vi "FaceGrabber.vi"() -> ()   [LabVIEW 2020]
uses:
  <vilib>/Utility/file.llb/Write Delimited Spreadsheet (string).vi
  <vilib>/vision/NI_Vision_Development_Module.lvlib
panel:
  in  "new table":bool
  in  "open table":bool
  out "Categories":string[](array[string])=["grooming", "aggression", "monkey_play", "group", "mating", "baby_monkey", "animals_playing", "hiding"]
  out "All Files in Dir":path[](array[path])
  out "data":cluster{"pictures":path, "table":path}
  in  "delete object":bool
  out "output array":string[][](array[string])
  in  "Table with results":path=path "C:/YandexDisk/MonkeysDatas/data/out/stimuli_set_lnv/area.csv"
  in  "save all":bool
  out "contours":T1(array[cluster])
  in  "category":u16(ring) items=["grooming", "aggression", "monkey_play", "group", "mating", "baby_monkey", "animals_playing", "hiding"]
  in  "add object":bool
  out "number of pictures":i32=120
  out "picture":i32
  in  "Stimuli Folder Path":path=path "C:/YandexDisk/MonkeysDatas/data/stimuli_set_lnv"
  in  "stop":bool
  in  "previous":bool
  in  "next":bool
  out "Image":T2(plugin-control)
  in  "baby/adult":bool=TRUE
  in  "face":bool=TRUE
  in  "animal":bool
  in  "monkey":bool=TRUE
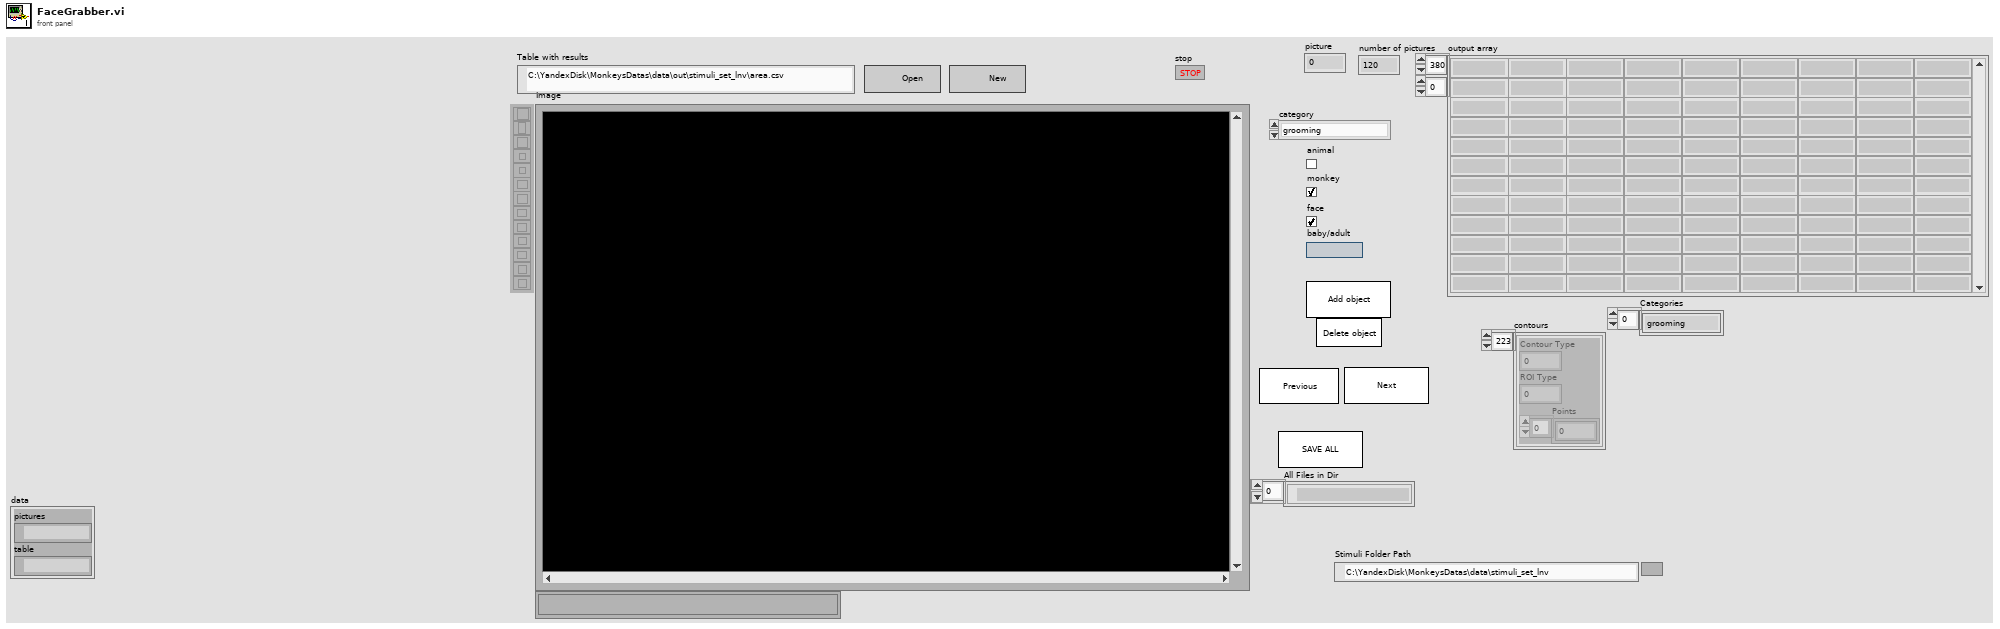
[diagram p1: front panel]
types:
  T1 = cluster{"Contour Type":u32, "ROI Type":u32, "Points":i32[]}[]
  T2 = typedef "IMAQ Image.ctl" = refnum<image>
  T3 = cluster{"stimuli pictures":path, "results table":path}
  T4 = cluster{"Stimuli Folder Path":path, "Table with results":path}
  T5 = cluster{"Global Rectangle":i32[], "Contours":cluster{"Contour Type":u32, "ROI Type":u32, "Points":i32[]}[]}
  T6 = typedef "Particle Parameters" = i32
  T7 = cluster{"Contour Type":u32, "ROI Type":u32, "Points":i32[]}
  T8 = cluster{"Stimuli Folder Path":path, "selected path":path}
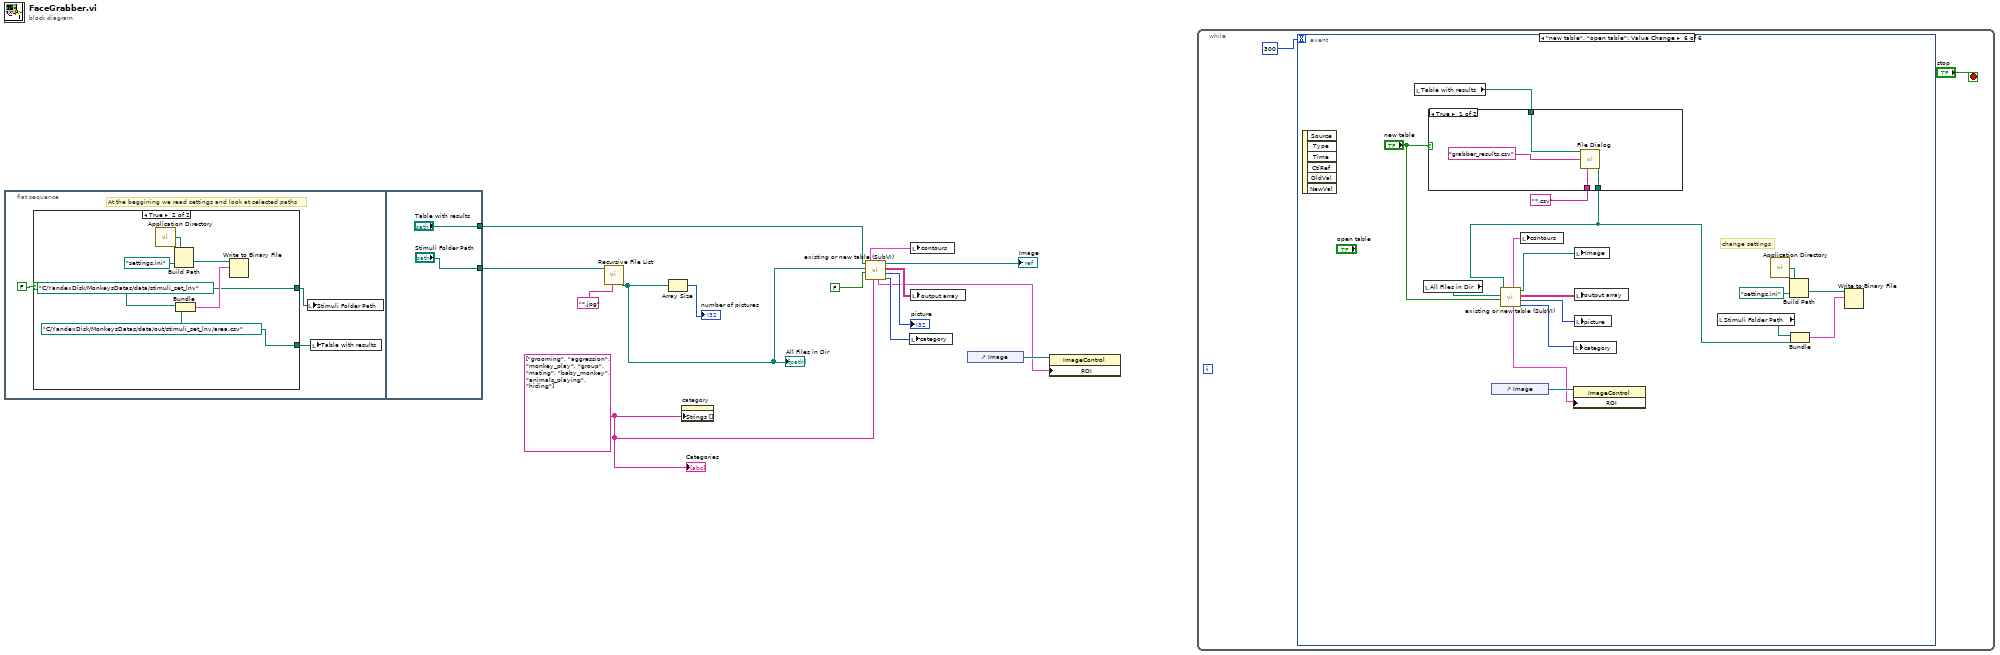
[diagram p0: block diagram]
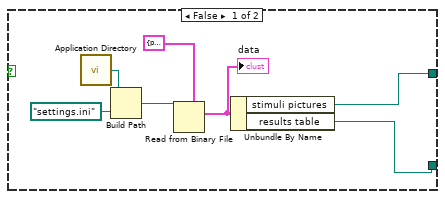
[diagram p2: hidden frame]
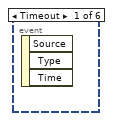
[diagram p3: hidden frame]
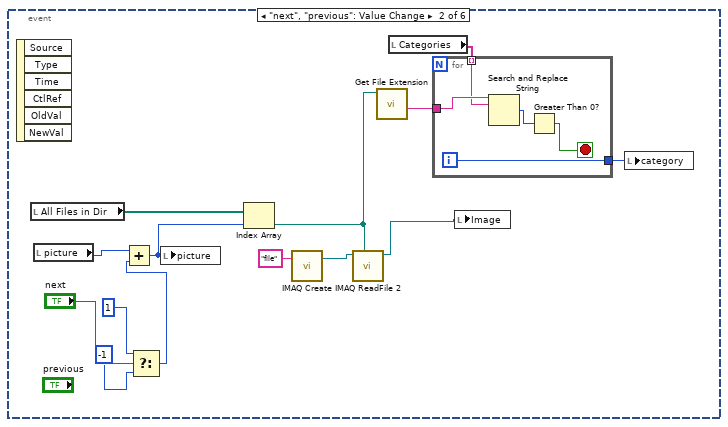
[diagram p4: hidden frame]
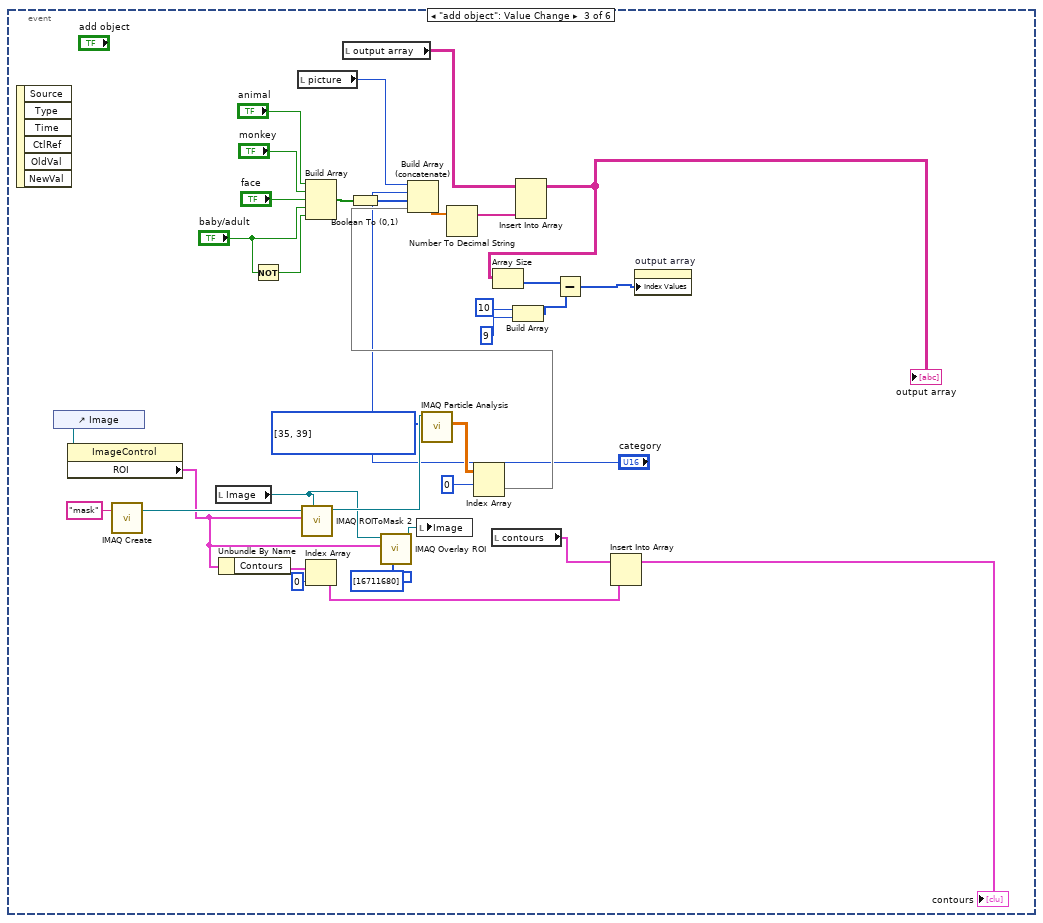
[diagram p5: hidden frame]
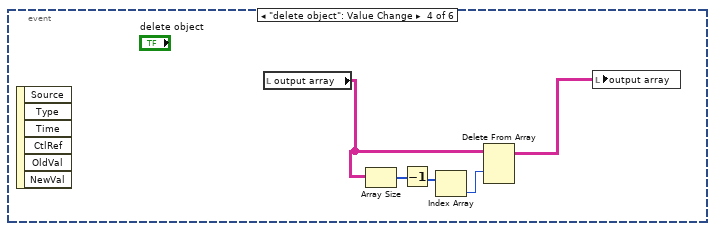
[diagram p6: hidden frame]
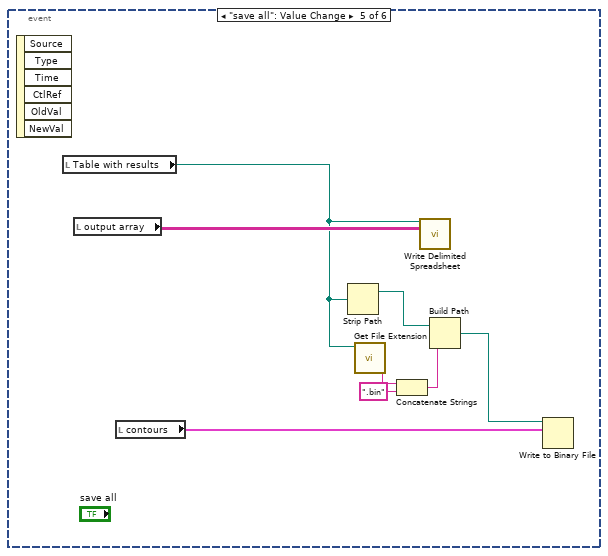
[diagram p7: hidden frame]
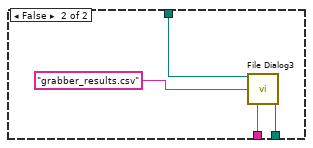
[diagram p8: hidden frame]
diagram:
  w3 = string[] ["grooming", "aggression", "monkey_play", "group", "mating", "baby_monkey", "animals_playing", "hiding"] ("Strings []")
  n1 = flat-sequence {
    tunnel: ["Table with results"] -> w2
    tunnel: ["Stimuli Folder Path"] -> w1
    frame #0 {
      # "At the beggining we read settings and look at selected paths"
      n2 = case shown="True" FALSE {
        tunnel: [w18 w26] -> w16
        tunnel: [w19 w25] -> w15
        frame False {
          n3 = call <vilib>:"Application Directory.vi"() -> ("Application Directory"=w22:path)
          n4 = Build Path(base path=w22, name or relative path=path "settings.ini") -> (appended path=w23:path)
          n5 = Read from Binary File(5:T3 {"stimuli pictures"=path "", "results table"=path ""} ("output cluster"), 11:w23) -> (2:w24:T3)  [unwired: 4 in, 3 out]
          "data" <- w24
          n6 = Unbundle By Name(w24) -> ("stimuli pictures"=w19:path, "results table"=w18:path)
        }
        frame True {
          w26 = path "C:/YandexDisk/MonkeysDatas/data/out/stimuli_set_lnv/area.csv" ("Table with results")
          w25 = path "C:/YandexDisk/MonkeysDatas/data/stimuli_set_lnv" ("Stimuli Folder Path")
          n7 = call <vilib>:"Application Directory.vi"() -> ("Application Directory"=w30:path)
          n8 = Build Path(base path=w30, name or relative path=path "settings.ini") -> (appended path=w28:path)
          n9 = Bundle("Stimuli Folder Path"=w25, "Table with results"=w26) -> (w27:T4)  [unwired: 1 in]
          n10 = Write to Binary File(file (use dialog)=w28, data=w27) -> ()  [unwired: 4 in, 3 out]
        }
      }
      n11 = local write "Stimuli Folder Path"(w15) -> ()
      n12 = local write "Table with results"(w16) -> ()
    }
    frame #1 {
    }
  }
  n13 = call <vilib>:"Recursive File List.vi"("pattern"="*.jpg", "Folder Path"=w1) -> ("All Files in Dir"=w4:path[])  [unwired: 5 in, 4 out]
  "All Files in Dir" <- w4
  n14 = Array Size(array=w4) -> (size(s)=→"number of pictures":i32)
  n15 = property on="category" class="Ring (strict)"("Strings []"=w3) -> ()  [unwired: 2 in, 2 out]
  n16 = call "existing or new table (SubVI).vi"("Categories (in)"=w3, "new table?"=FALSE, "All Files in Dir (in)"=w4, "table"=w2) -> ("category"=w6:i32, "picture"=→"picture":i32, "text table"=w7:string[][], "Refnum out"=→"Image":T2, "ROI"=w5:T5, "contours"=w8:T1)  [unwired: 2 in]
  n17 = local write "category"(w6) -> ()
  n18 = local write "contours"(w8) -> ()
  n19 = local write "output array"(w7) -> ()
  n20 = control-ref of="Image"() -> (w12:refnum<vi>)
  n21 = property class="ImageControl"(reference=w12, "ROI"=w5) -> ()  [unwired: 1 in, 2 out]
  n22 = while {
    stop <- "stop" stop-if-true
    n23 = event shown="[5] \"new table\", \"open table\": Value Change" {
      selector: _ -> [_ _ _ _ _ _]
      dyn-events: _ -> [_ _ _ _ _ _]
      timeout: 300 -> [_ _ _ _ _ _]
      event Timeout {
        n24 = event-data() -> ()  [unwired: 1 in, 3 out]
      }
      event "next", "previous": Value Change {
        n25 = event-data() -> ()  [unwired: 1 in, 6 out]
        n26 = local read "All Files in Dir"() -> (w37:path[])
        n27 = local read "picture"() -> (w36:i32)
        n28 = Select(t=1 ("y"), s="next", f=-1 ("y")) -> (s? t:f=w42:i32)
        n29 = Add(x=w36, y=w42) -> (x+y=w41:i32)
        n30 = local write "picture"(w41) -> ()
        n31 = Index Array(array=w37, index=w41) -> (element=w40:path)
        n32 = call "IMAQ Create"("Image Name"="file") -> ("New Image"=w48:T2)  [unwired: 4 in, 1 out]
        n33 = call "IMAQ ReadFile 2"("File Path"=w40, "Image"=w48) -> ("Image Out"=w46:T2)  [unwired: 5 in, 4 out]
        n34 = call <vilib>:"Get File Extension.vi"("file"=w40) -> ("filename without extension"=w39:string)  [unwired: 6 in, 4 out]
        n35 = local read "Categories"() -> (w35:string[])
        n36 = for {
          tunnel: w35 -> [w52] mode=indexing
          tunnel: w39 -> [w53]
          tunnel: [w49] -> w38
          i -> [w49]
          stop <- w50 stop-if-true
          n37 = Search and Replace String(input string=w53, search string=w52) -> (number of replacements=w51:i32)  [unwired: 6 in, 3 out]
          n38 = Greater Than 0?(x=w51) -> (x > 0?=w50:bool)
        }
        n39 = local write "Image"(w46) -> ()
        n40 = local write "category"(w38) -> ()
      }
      event "add object": Value Change {
        w79 = T6[] [35, 39] items=["Center of Mass X", "Center of Mass Y", "First Pixel X", "First Pixel Y", "Bounding Rect Left", "Bounding Rect Top", "Bounding Rect Right", "Bounding Rect Bottom", "Max Feret Diameter Start X", "Max Feret Diameter Start Y", "Max Feret Diameter End X", "Max Feret Diameter End Y", "Max Horiz. Segment Length Left", "Max Horiz. Segment Length Right", "Max Horiz. Segment Length Row", "-", "Bounding Rect Width", "Bounding Rect Height", "Bounding Rect Diagonal", "Perimeter", "Convex Hull Perimeter", "Holes' Perimeter", "Max Feret Diameter", "Equivalent Ellipse Major Axis", "Equivalent Ellipse Minor Axis", "Equivalent Ellipse Minor Axis (Feret)", "Equivalent Rect Long Side", "Equivalent Rect Short Side", "Equivalent Rect Diagonal", "Equivalent Rect Short Side (Feret)", "Average Horiz. Segment Length", "Average Vert. Segment Length", "Hydraulic Radius", "Waddel Disk Diameter", "-", "Area", "Holes' Area", "Particle & Holes' Area", "Convex Hull Area", "Image Area", "-", "Number of Holes", "Number of Horiz. Segments", "Number of Vert. Segments", "-", "Orientation", "Max Feret Diameter Orientation", "-", "% Area/Image Area", "% Area/(Particle & Holes' Area)", "Ratio of Equivalent Ellipse Axes", "Ratio of Equivalent Rect Sides", "-", "Elongation Factor", "Compactness Factor", "Heywood Circularity Factor", "Type Factor", "-", "Sum X", "Sum Y", "Sum XX", "Sum XY", "Sum YY", "Sum XXX", "Sum XXY", "Sum XYY", "Sum YYY", "-", "Moment of Inertia XX", "Moment of Inertia XY", "Moment of Inertia YY", "Moment of Inertia XXX", "Moment of Inertia XXY", "Moment of Inertia XYY", "Moment of Inertia YYY", "Norm. Moment of Inertia XX", "Norm. Moment of Inertia XY", "Norm. Moment of Inertia YY", "Norm. Moment of Inertia XXX", "Norm. Moment of Inertia XXY", "Norm. Moment of Inertia XYY", "Norm. Moment of Inertia YYY", "Hu Moment 1", "Hu Moment 2", "Hu Moment 3", "Hu Moment 4", "Hu Moment 5", "Hu Moment 6", "Hu Moment 7"] ("Pixel Measurements")
        n41 = event-data() -> ()  [unwired: 1 in, 6 out]
        n42 = control-ref of="Image"() -> (w77:refnum<vi>)
        n43 = property class="ImageControl"(reference=w77) -> ("ROI"=w59:T5)  [unwired: 1 in, 2 out]
        n44 = call "IMAQ Create"("Image Name"="mask") -> ("New Image"=w82:T2)  [unwired: 4 in, 1 out]
        n45 = local read "Image"() -> (w60:T2)
        n46 = Unbundle By Name(w59) -> ("Contours"=w76:T1)
        n47 = Not(x="baby/adult") -> (.not. x?=w55:bool)
        n48 = local read "picture"() -> (w54:i32)
        n49 = call "IMAQ ROIToMask 2"("Image Model"=w60, "ROI Descriptor"=w59, "Image"=w82) -> ("Image Out"=w83:T2)  [unwired: 6 in, 2 out]
        n50 = Build Array("animal", "monkey", "face", "baby/adult", w55) -> (w87:bool[])
        n51 = Index Array(array=w76, index=0) -> (element=w71:T7)
        n52 = local read "output array"() -> (w74:string[][])
        n53 = Boolean To (0,1)(Boolean=w87) -> (0, 1=w88:i16[])
        n54 = call "IMAQ Overlay ROI"("Colors (Green)"=u32[] [16711680], "ROI Descriptor"=w59, "Image"=w60) -> ("Image Out"=w58:T2)  [unwired: 7 in, 1 out]
        n55 = local write "Image"(w58) -> ()
        n56 = call "IMAQ Particle Analysis"("Pixel Measurements"=w79, "Image"=w83) -> ("Particle Measurements (Pixels)"=w81:dbl[][])  [unwired: 4 in, 5 out]
        n57 = Index Array(array=w81, index (row)=0 ("disabled index (col)")) -> (element=w78:dbl[])  [unwired: 1 in]
        n58 = Build Array (concatenate)(w54, "category", w88, w78) -> (w73:dbl[])
        n59 = Number To Decimal String(number=w73) -> (decimal integer string=w67:string[])  [unwired: 1 in]
        n60 = local read "contours"() -> (w69:T1)
        n61 = Build Array(10, 9) -> (w64:i32[])
        n62 = Insert Into Array(array=w74, new element=w67) -> (w66:string[][])  [unwired: 2 in]
        "output array" <- w66
        n63 = Array Size(array=w66) -> (size(s)=w65:i32[])
        n64 = Subtract(x=w65, y=w64) -> (x-y=w63:i32[])
        n65 = Insert Into Array(array=w69, new element=w71) -> (→"contours":T1)  [unwired: 1 in]
        n66 = property on="output array" class="Arr (strict)"("Index Values"=w63) -> ()  [unwired: 2 in, 2 out]
      }
      event "delete object": Value Change {
        n67 = event-data() -> ()  [unwired: 1 in, 6 out]
        n68 = local read "output array"() -> (w90:string[][])
        n69 = Array Size(array=w90) -> (size(s)=w91:i32[])
        n70 = Decrement(x=w91) -> (x-1=w92:i32[])
        n71 = Index Array(array=w92) -> (element=w93:i32)  [unwired: 1 in]
        n72 = Delete From Array(array=w90, index (row)=w93) -> (array with subset deleted=w89:string[][])  [unwired: 2 in, 1 out]
        n73 = local write "output array"(w89) -> ()
      }
      event "save all": Value Change {
        n74 = event-data() -> ()  [unwired: 1 in, 6 out]
        n75 = local read "Table with results"() -> (w94:path)
        n76 = local read "output array"() -> (w95:string[][])
        n77 = local read "contours"() -> (w101:T1)
        n78 = Strip Path(path=w94) -> (stripped path=w97:path)  [unwired: 1 out]
        n79 = call <vilib>:"Get File Extension.vi"("file"=w94) -> ("filename without extension"=w100:string)  [unwired: 6 in, 4 out]
        n80 = Concatenate Strings(w100, ".bin" ("string")) -> (w98:string)
        n81 = call-poly <vilib>:"Write Delimited Spreadsheet.vi"("file path (dialog if empty)"=w94, "2D data"=w95) -> ()  [unwired: 12 in, 2 out]
        n82 = Build Path(base path=w97, name or relative path=w98) -> (appended path=w96:path)
        n83 = Write to Binary File(file (use dialog)=w96, data=w101) -> ()  [unwired: 4 in, 3 out]
      }
      event "new table", "open table": Value Change {
        # "change settings"
        n84 = event-data() -> ()  [unwired: 1 in, 6 out]
        n85 = local read "Table with results"() -> (w109:path)
        n86 = local read "All Files in Dir"() -> (w110:path[])
        n87 = case shown="True" "new table" {
          tunnel: [w122 w126] -> w102
          tunnel: w109 -> [w120 w124]
          tunnel: "*.csv" ("pattern (all files)") -> [w119 w123]
          frame True {
            n88 = call "File Dialog"("start path"=w120, "default name"="grabber_results.csv", "pattern (all files)"=w119) -> ("selected path"=w122:path)  [unwired: 9 in, 3 out]
          }
          frame False {
            n89 = call "File Dialog3"("start path"=w124, "default name"="grabber_results.csv", "pattern (all files)"=w123) -> ("selected path"=w126:path)  [unwired: 9 in, 3 out]
          }
        }
        n90 = control-ref of="Image"() -> (w107:refnum<vi>)
        n91 = call "existing or new table (SubVI).vi"("new table?"="new table", "All Files in Dir (in)"=w110, "table"=w102) -> ("category"=w112:i32, "picture"=w113:i32, "text table"=w114:string[][], "Refnum out"=w111:T2, "ROI"=w106:T5, "contours"=w105:T1)  [unwired: 3 in]
        n92 = local write "contours"(w105) -> ()
        n93 = local write "category"(w112) -> ()
        n94 = property class="ImageControl"(reference=w107, "ROI"=w106) -> ()  [unwired: 1 in, 2 out]
        n95 = local write "output array"(w114) -> ()
        n96 = local write "picture"(w113) -> ()
        n97 = local write "Image"(w111) -> ()
        n98 = local read "Stimuli Folder Path"() -> (w103:path)
        n99 = call <vilib>:"Application Directory.vi"() -> ("Application Directory"=w115:path)
        n100 = Build Path(base path=w115, name or relative path=path "settings.ini") -> (appended path=w117:path)
        n101 = Bundle("Stimuli Folder Path"=w103, "selected path"=w102) -> (w118:T8)  [unwired: 1 in]
        n102 = Write to Binary File(file (use dialog)=w117, data=w118) -> ()  [unwired: 4 in, 3 out]
      }
    }
  }
  "Categories" <- w3
